vi "new Segment.vi"(6 "error in (no error)":errorcluster, 9 "Data":T1={"Report.lvclass"=refnum, "test"="", "last State"=enum."Initialize", "test ID"=0, "parameter"=[], "EMTestCWS500N.lvclass"=refnum, "CEG4500.lvclass"=refnum, "Tektronix RSA5106A.lvclass"=refnum, "erfolgreich"=FALSE, "log"="", "Kommentar"="", "Device Enum"=enum."emTestCWS500N", "Test Enum"=enum."HF-Felder", "debug"=FALSE}) -> (0 "error out":errorcluster, 1 "abbrechen":bool, 2 "Segment.lvclass 2":refnum<class "Segment.lvclass">)   [LabVIEW 2013, in "DataCreation.lvlib"]
uses:
  lib/DataCreation.lvlib
  Main/controls/Data.ctl
  classes/Datastructure/Report/Report.lvclass
  classes/Devices/emTestCWS500N/EMTestCWS500N.lvclass
  classes/Devices/CEG4500/CEG4500.lvclass
  classes/Devices/Tektronix RSA5106A/Tektronix RSA5106A.lvclass
  Main/controls/State.ctl
  classes/Devices/DeviceInterface/Devices.ctl
  classes/Tests/TestInterface/Tests.ctl
  classes/Datastructure/Segment/Segment.lvclass
  classes/Datastructure/Test/Test.lvclass
  classes/Datastructure/Image/img.lvclass
  lib/TreeRepresentation.lvlib
panel:
  in  "number of pictures":i32
  in  "Tab Control":enum32{"neues Segment", "Daten"}(tab)
  in  "Cancel Button":bool
  in  "Tree 2":string(tree)
  out "Test":string
  in  "OK Button":bool
  in  "Add picture":bool
  in  "Kommentar":string
  in  "Segement Name":string
  in  "Parameter":string[][](table)
  in  "Tree":string(tree)
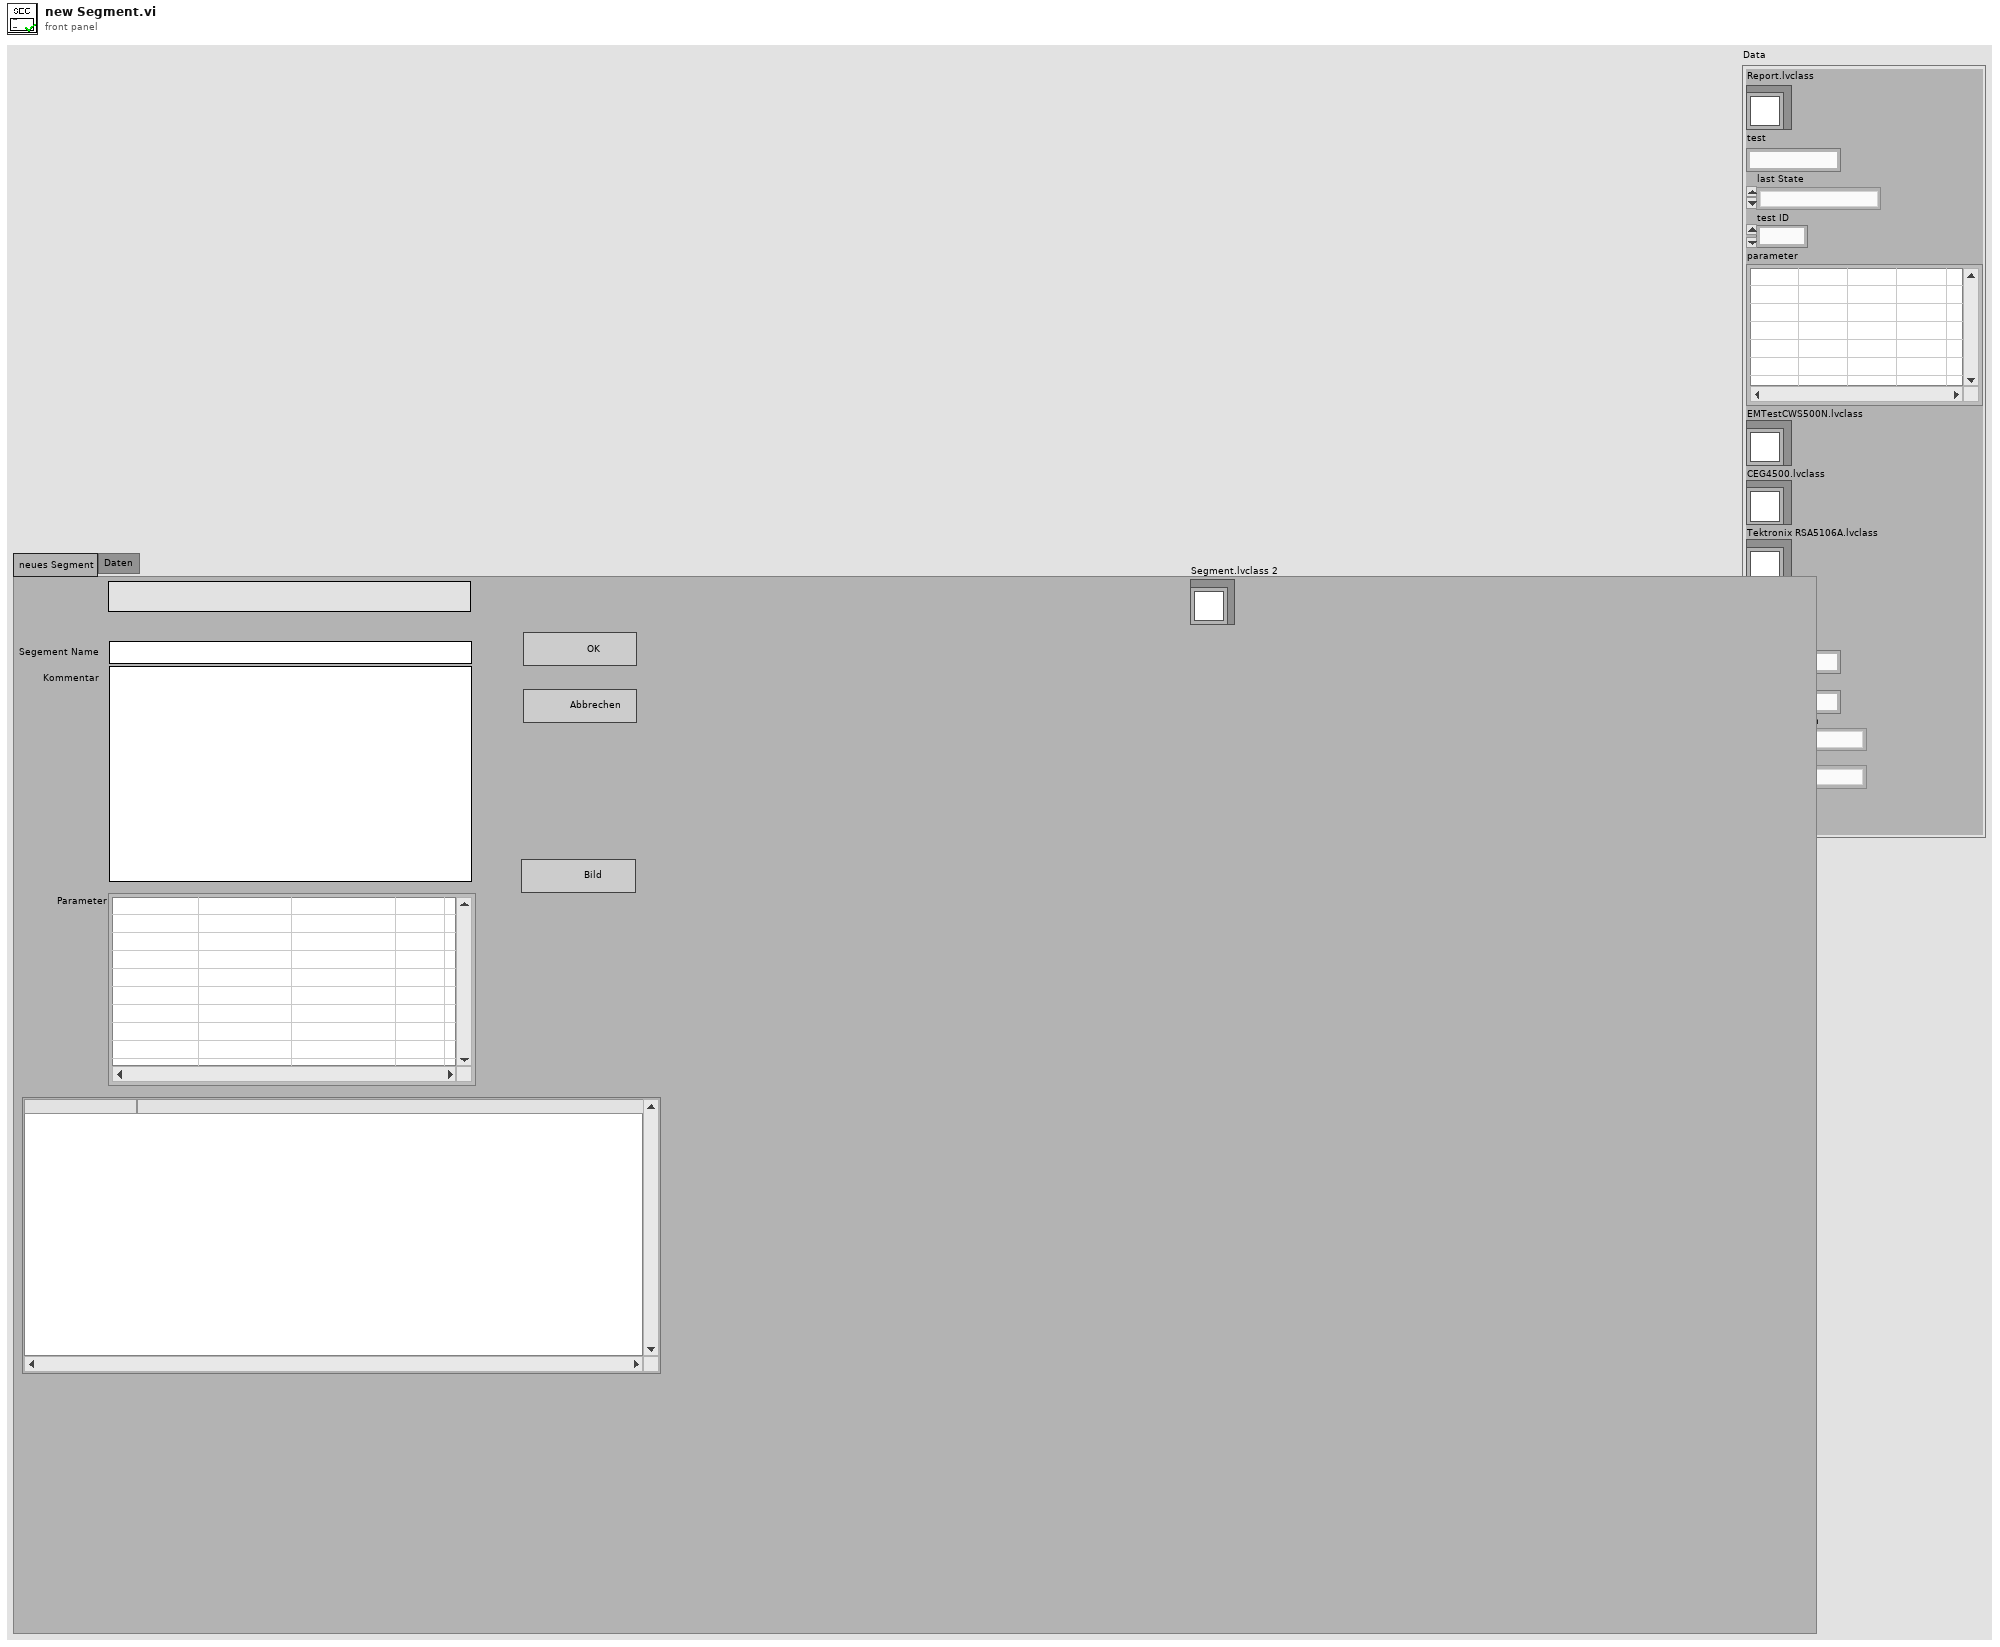
[diagram p1: front panel]
types:
  T1 = typedef "Data.ctl" = cluster{"Report.lvclass":refnum<class "Report.lvclass">, "test":string, "last State":T2, "test ID":i32, "parameter":string[][], "EMTestCWS500N.lvclass":refnum<class "EMTestCWS500N.lvclass">, "CEG4500.lvclass":refnum<class "CEG4500.lvclass">, "Tektronix RSA5106A.lvclass":refnum<class "Tektronix RSA5106A.lvclass">, "erfolgreich":bool, "log":string, "Kommentar":string, "Device Enum":T3, "Test Enum":T4, "debug":bool}
  T2 = typedef "State.ctl" = enum16{"create Pdf", "load Report", "save Report", "do Test", "CDN Kalibrierung", "enter Report Parameters", "new Test", "Protokoll", "read Tree", "update Tree", "Fehler", "Initialize", "Wait for Event", "Exit"}
  T3 = typedef "Devices.ctl" = enum16{"unbekannt", "Tektronix RSA5106A", "emTestCWS500N", "CEG-4500"}
  T4 = typedef "Tests.ctl" = enum16{"unbekannt", "Störaussendung", "Burst", "ESD", "Surge", "Spannungseinbruch", "HF-Felder"}
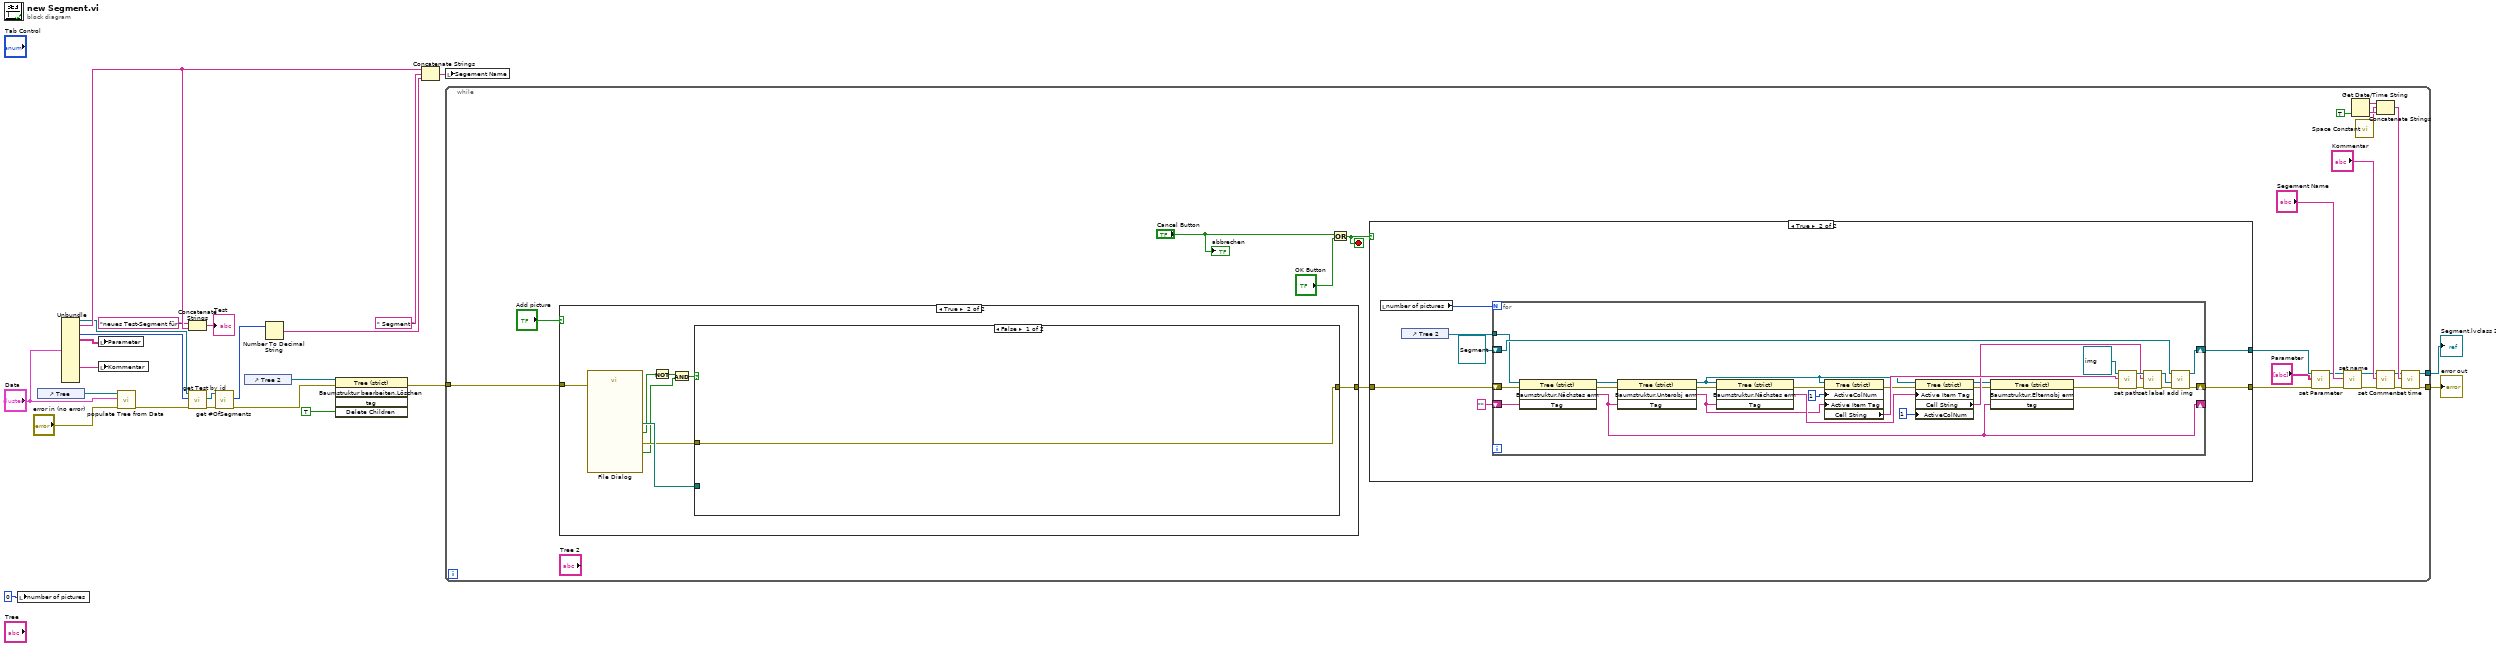
[diagram p0: block diagram]
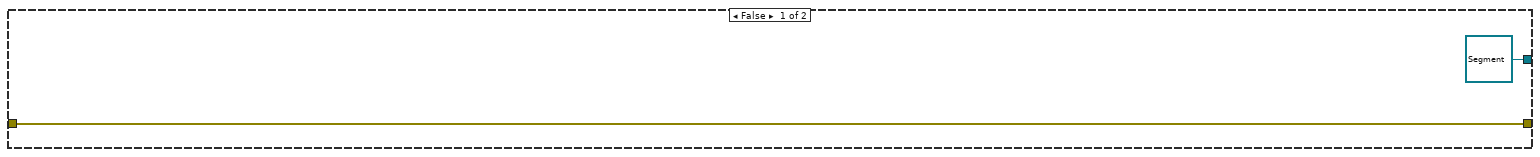
[diagram p2: hidden frame]
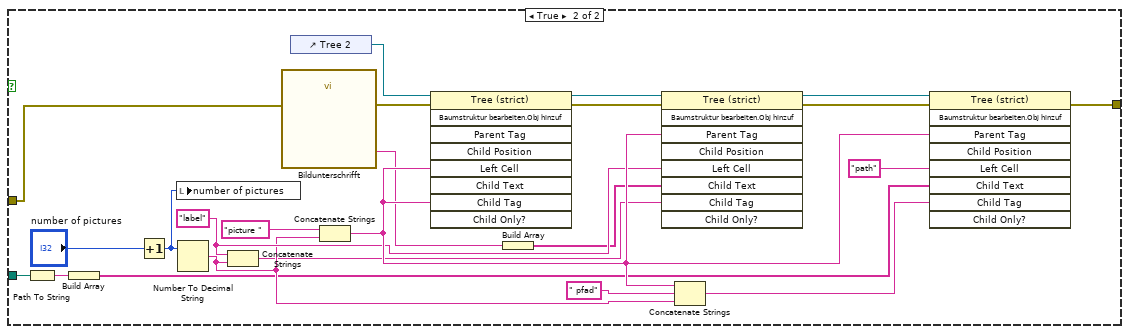
[diagram p4: hidden frame]
diagram:
  n1 = local write "number of pictures"(0 ("number of pictures")) -> ()
  n2 = control-ref of="Tree"() -> (w24:refnum<vi>)
  n3 = Unbundle("Data") -> ("Report.lvclass"=w19:refnum<class "Report.lvclass">, "test"=w21:string, "test ID"=w20:i32, "parameter"=w1:string[][], "Kommentar"=w5:string)  [unwired: 9 out]
  n4 = local write "Parameter"(w1) -> ()
  n5 = local write "Kommentar"(w5) -> ()
  n6 = call "populate Tree from Data.vi"("error in (no error)"="error in (no error)", "Data"="Data", "reference"=w24) -> ("error out"=w18:errorcluster)  [unwired: 6 in]
  n7 = Concatenate Strings("neues Test-Segment für ", w21) -> (→"Test":string)
  n8 = call-dynamic "get Test by id.vi"("error in (no error)"=w18, "id"=w20, "Report (Eingang)"=w19) -> ("error out"=w15:errorcluster, "Test.lvclass"=w17:refnum<class "Test.lvclass">)  [unwired: 4 in, 3 out]
  n9 = call-dynamic "get #OfSegments.vi"("error in (no error)"=w15, "Test (Eingang)"=w17) -> ("error out"=w9:errorcluster, "#OfSegments"=w16:u32)  [unwired: 7 in, 1 out]
  n10 = control-ref of="Tree 2"() -> (w7:refnum<vi>)
  n11 = Number To Decimal String(number=w16) -> (decimal integer string=w12:string)  [unwired: 1 in]
  n12 = invoke class="Tree (strict)" method="Baumstruktur bearbeiten.Löschen"(reference=w7, error in=w9, "Delete Children"=TRUE ("Unterobjekte löschen?")) -> (error out=w8:errorcluster)  [unwired: 2 in, 4 out]
  n13 = Concatenate Strings(w21, " Segment ", w12) -> (w3:string)
  n14 = local write "Segement Name"(w3) -> ()
  n15 = while {
    tunnel: w8 -> [w46]
    tunnel: [w34] -> w11
    tunnel: [w33] -> w10
    stop <- w26 stop-if-true
    n16 = case shown="True" "Add picture" {
      tunnel: [w85 w91] -> w47
      tunnel: w46 -> [w85 w90]
      frame False {
      }
      frame True {
        n17 = call "File Dialog"("error in"=w90) -> ("selected path"=w93:path, "exists"=w86:bool, "cancelled"=w89:bool, "error out"=w92:errorcluster)  [unwired: 11 in]
        n18 = Not(x=w89) -> (.not. x?=w87:bool)
        n19 = And(x=w87, y=w86) -> (x .and. y?=w88:bool)
        n20 = case shown="False" w88 {
          tunnel: w93 -> [_ w108]
          tunnel: w92 -> [w94 w103]
          tunnel: [w94 w95] -> w91
          frame False {
          }
          frame True {
            w111 = "label" ("Left Cell String")
            n21 = Path To String(path=w108) -> (string=w104:string)
            n22 = Build Array(w104) -> (w107:string[])
            n23 = Increment(x="number of pictures") -> (x+1=w99:i32)
            n24 = local write "number of pictures"(w99) -> ()
            n25 = Number To Decimal String(number=w99) -> (decimal integer string=w110:string)  [unwired: 1 in]
            n26 = Concatenate Strings(w111, w110) -> (w109:string)
            n27 = call "Bildunterschrifft"("error in (no error)"=w103) -> ("Bildunterschrifft"=w102:string, "error out"=w98:errorcluster)  [unwired: 16 in, 1 out]
            n28 = control-ref of="Tree 2"() -> (w117:refnum<vi>)
            n29 = Concatenate Strings("picture " ("Left Cell String"), w110) -> (w112:string)
            n30 = invoke class="Tree (strict)" method="Baumstruktur bearbeiten.Obj hinzuf"(reference=w117, error in=w98, "Left Cell"=w112, "Child Tag"=w112) -> (reference out=w106:refnum<vi>, error out=w97:errorcluster)  [unwired: 5 in, 7 out]
            n31 = Build Array(w102) -> (w101:string[])
            n32 = invoke class="Tree (strict)" method="Baumstruktur bearbeiten.Obj hinzuf"(reference=w106, error in=w97, "Parent Tag"=w112, "Left Cell"=w111, "Child Text"=w101, "Child Tag"=w109) -> (reference out=w105:refnum<vi>, error out=w96:errorcluster)  [unwired: 3 in, 7 out]
            n33 = Concatenate Strings(w112, " pfad", w110) -> (w114:string)
            n34 = invoke class="Tree (strict)" method="Baumstruktur bearbeiten.Obj hinzuf"(reference=w105, error in=w96, "Parent Tag"=w112, "Left Cell"="path" ("Left Cell String"), "Child Text"=w107, "Child Tag"=w114) -> (error out=w95:errorcluster)  [unwired: 3 in, 8 out]
          }
        }
      }
    }
    n35 = Or(x="Cancel Button", y="OK Button") -> (x .or. y?=w26:bool)
    n36 = case shown="True" w26 {
      tunnel: [refnum<class "Segment.lvclass"> refnum ("Segment.lvclass") w57] -> w32
      tunnel: [w49 w56] -> w31
      tunnel: w47 -> [w49 w55]
      frame False {
      }
      frame True {
        n37 = local read "number of pictures"() -> (w52:i32)
        n38 = control-ref of="Tree 2"() -> (w53:refnum<vi>)
        n39 = for {
          N: w52 -> [_]
          tunnel: w53 -> [w63]
          shift-right: [w75] -> w57
          shift-left: refnum<class "Segment.lvclass"> refnum ("Segment.lvclass") -> [w83]
          shift-right: [w68] -> w56
          shift-left: w55 -> [w67]
          shift-right: [w62] -> _
          shift-left: "" ("Navigate Tree:Get Next Item") -> [w61]
          n40 = invoke class="Tree (strict)" method="Baumstruktur.Nächstes erm"(reference=w63, error in=w67, "Tag"=w61) -> (reference out=w84:refnum<vi>, error out=w74:errorcluster, "Navigate Tree:Get Next Item"=w62:string)  [unwired: 1 in, 1 out]
          n41 = invoke class="Tree (strict)" method="Baumstruktur.Unterobj erm"(reference=w84, error in=w74, "Tag"=w62) -> (reference out=w79:refnum<vi>, error out=w73:errorcluster, "Navigate Tree:Get Child"=w60:string)  [unwired: 1 in, 1 out]
          n42 = invoke class="Tree (strict)" method="Baumstruktur.Nächstes erm"(reference=w79, error in=w73, "Tag"=w60) -> (error out=w72:errorcluster, "Navigate Tree:Get Next Item"=w78:string)  [unwired: 1 in, 2 out]
          n43 = property class="Tree (strict)"(reference=w79, error in=w72, "ActiveColNum"=1 ("Active Cell:Active Column Number"), "Active Item Tag"=w60) -> (error out=w71:errorcluster, "Cell String"=w80:string)  [unwired: 1 out]
          n44 = property class="Tree (strict)"(reference=w79, error in=w71, "Active Item Tag"=w78, "ActiveColNum"=1 ("Active Cell:Active Column Number")) -> (reference out=w64:refnum<vi>, error out=w59:errorcluster, "Cell String"=w77:string)
          n45 = invoke class="Tree (strict)" method="Baumstruktur.Elternobj erm"(reference=w64, error in=w59, "tag"=w62) -> (error out=w58:errorcluster)  [unwired: 1 in, 3 out]
          n46 = call-dynamic "set path.vi"("error in (no error)"=w58, "path"=w80, "img (Eingang)"=refnum<class "img.lvclass"> refnum ("img.lvclass")) -> ("error out"=w70:errorcluster, "img (Ausgang)"=w82:refnum<class "img.lvclass">)  [unwired: 7 in]
          n47 = call-dynamic "set label.vi"("error in (no error)"=w70, "label"=w77, "img (Eingang)"=w82) -> ("error out"=w69:errorcluster, "img (Ausgang)"=w76:refnum<class "img.lvclass">)  [unwired: 7 in]
          n48 = call-dynamic "add img.vi"("error in (no error)"=w69, "img.lvclass"=w76, "Segment (Eingang)"=w83) -> ("error out"=w68:errorcluster, "Segment (Ausgang)"=w75:refnum<class "Segment.lvclass">)  [unwired: 6 in]
        }
      }
    }
    n49 = call-dynamic "set Parameter.vi"("error in (no error)"=w31, "Parameter"="Parameter", "Segment (Eingang)"=w32) -> ("error out"=w28:errorcluster, "Segment (Ausgang)"=w29:refnum<class "Segment.lvclass">)  [unwired: 7 in]
    n50 = call-dynamic "set name.vi"("error in (no error)"=w28, "name"="Segement Name", "Segment (Eingang)"=w29) -> ("error out"=w35:errorcluster, "Segment (Ausgang)"=w38:refnum<class "Segment.lvclass">)  [unwired: 7 in]
    n51 = Get Date/Time String(want seconds? (F)=TRUE) -> (date string=w42:string, time string=w43:string)  [unwired: 2 out]
    n52 = call <vilib>:"Space Constant.vi"() -> ("String"=w41:string)
    n53 = Concatenate Strings(w42, w41, w43) -> (w39:string)
    n54 = call-dynamic "set Comment.vi"("error in (no error)"=w35, "Comment"="Kommentar", "Segment (Eingang)"=w38) -> ("error out"=w36:errorcluster, "Segment (Ausgang)"=w37:refnum<class "Segment.lvclass">)  [unwired: 7 in]
    n55 = call-dynamic "set time.vi"("error in (no error)"=w36, "time"=w39, "Segment (Eingang)"=w37) -> ("error out"=w34:errorcluster, "Segment (Ausgang)"=w33:refnum<class "Segment.lvclass">)  [unwired: 7 in]
    "abbrechen" <- "Cancel Button"
  }
  "error out" <- w11
  "Segment.lvclass 2" <- w10
